vi "Init Queues.vi"(8 "error in (no error) in":errorcluster) -> (0 "error out":errorcluster, 3 "Queues":T1)   [LabVIEW 2017]
uses:
  Controls/Queues.ctl
  Controls/Frame Grabber State.ctl
  Controls/Optitrack State.ctl
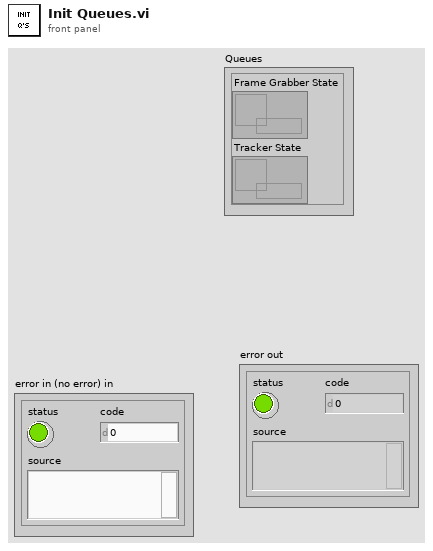
[diagram p1: front panel]
types:
  T1 = typedef "Queues.ctl" = cluster{"Frame Grabber State":refnum<queue>, "Tracker State":refnum<queue>}
  T2 = typedef "Optitrack State.ctl" = enum16{"Wait", "Init", "Grab Rigid Body Data", "Error Handling", "Shutdown"}
  T3 = typedef "Frame Grabber State.ctl" = enum16{"Wait", "Init", "Update Geometry", "Set Crop ROI", "Clear Crop ROI", "Configure Live", "Configure Recording", "Start Playback", "Grab Live Frame", "Record Frame", "Playback Frame", "Unconfigure Live", "End Recording", "Stop Playback", "Error Handling", "Shutdown"}
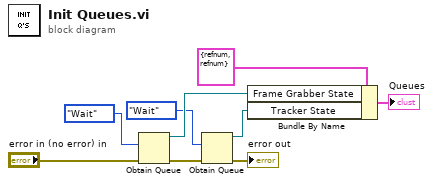
[diagram p0: block diagram]
diagram:
  n1 = Obtain Queue(element data type=Frame_Grabber_State."Wait", error in (no error)="error in (no error) in") -> (queue out=w7:refnum<queue>, error out=w3:errorcluster)  [unwired: 3 in, 1 out]
  n2 = Obtain Queue(element data type=Optitrack_State."Wait" ("OptiTrack State"), error in (no error)=w3) -> (queue out=w1:refnum<queue>, error out=→"error out":errorcluster)  [unwired: 3 in, 1 out]
  n3 = Bundle By Name(cluster=T1 {"Frame Grabber State"=refnum, "Tracker State"=refnum}, "Frame Grabber State"=w7, "Tracker State"=w1) -> (→"Queues":T1)
